vi "Main Page.vi"(8 "error in (no error)":errorcluster, 11 "Node Ptr":T1 format="%.0x") -> (0 "error out":errorcluster)   [LabVIEW 2018, in "Instrument Addon System Explorer.lvlib"]
uses:
  Instrument Addon System Explorer.lvlib
  <vilib>/NI Veristand/Custom Device API/Custom Device Item Ref.ctl
  Addon Shared/Types/FG Control.ctl
  Addon Shared/SubVIs/Constants.vi
  <vilib>/NI/NI VeriStand Advanced SysDef API/SysDef API/SysDef.Property.Get.vi
  <vilib>/NI/NI VeriStand Advanced SysDef API/_SubVIs/SysDef.Property.Get.String.vi
  <vilib>/NI/NI VeriStand Advanced SysDef API/SysDef API/SysDef.Property.Set.vi
  <vilib>/NI/NI VeriStand Advanced SysDef API/_SubVIs/SysDef.Property.Set.String.vi
  <vilib>/Utility/LVClass/Get LV Class Default Value.vi
  Support Libraries/Protocols.lvlibp/TCP/Settings Page.vi
  <vilib>/NI Veristand/Custom Device API/NI VeriStand - Get Item Property.vi
  <vilib>/NI Veristand/Custom Device API/Get Item Property (Boolean).vi
  <vilib>/NI Veristand/Custom Device API/Get Item Property (U32).vi
  <vilib>/NI Veristand/Custom Device API/Get Item Property (String).vi
  <vilib>/NI Veristand/Custom Device API/NI VeriStand - Set Item Property.vi
  <vilib>/NI Veristand/Custom Device API/Set Item Property (Boolean).vi
  <vilib>/NI Veristand/Custom Device API/Set Item Property (U32).vi
  <vilib>/NI Veristand/Custom Device API/Set Item Property (String).vi
  Support Libraries/Protocols.lvlibp/Protocol Parent/Protocol Parent.lvclass
  <vilib>/NI Veristand/Custom Device API/Custom Device API.lvlib
  Addon Shared/Instrument Addon Shared.lvlib
  APIs/Scripting API/Instrument Addon Scripting API.lvlib
  Support Libraries/Protocols.lvlibp/TCP/TCP.lvclass
panel:
  out "Version":string
  in  "PCL Decimation":u32=1 min=1 max=10000 step=1
  in  "Protocol":string(combo)
  in  "SHDocVw.IWebBrowser":refnum<k7>(container)
  in  "Header":cluster{"Section Name":string}={"Section Name"="Addon Settings"}
  in  "Description":string
  in  "Name":string
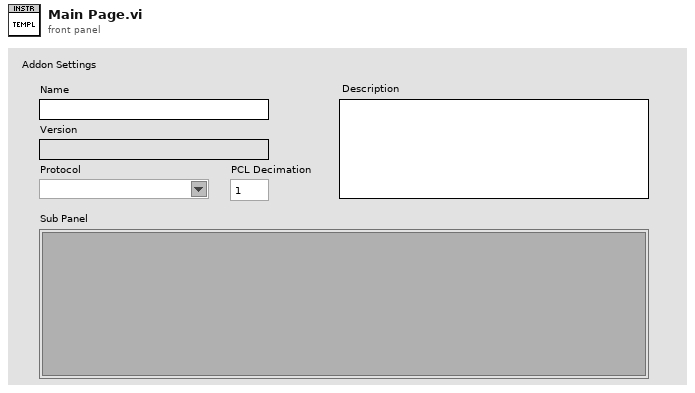
[diagram p1: front panel]
types:
  T1 = typedef "Custom Device API.lvlib/Custom Device Item Ref.ctl" = u64
  T2 = typedef "Custom Device API.lvlib/Custom Device Item Info.ctl" = cluster{"Name":string, "Is Channel":bool, "GUID":string, "Is Waveform":bool}
  T3 = typedef "Instrument Addon Shared.lvlib/FG Control.ctl" = enum16{"Get", "Set"}
  T4 = typedef "Custom Device API.lvlib/Custom Device Commands.ctl" = enum16{"Default", "Item renamed", "Shutdown", "Dynamic button pressed"}
  T5 = typedef "Protocols.lvlibp/Protocol Parent.lvclass/Base Protocol Type.ctl" = enum16{"RS-XXX", "VISA", "TCPIP", "UDP", "GPIB ConvBox"}
  T6 = typedef "Instrument Addon Shared.lvlib/VISA Settings.ctl" = cluster{"VISA Resource":string, "Enable Termination Character":bool, "Termination Character":u8, "Timeout":u32, "Append Write Termination Character":bool}
  T7 = typedef "Instrument Addon Shared.lvlib/TCPIP Settings.ctl" = cluster{"IP Address":string, "Port":u16}
  T8 = typedef "Instrument Addon Shared.lvlib/UDP Settings.ctl" = cluster{"Local IP Address":string, "Local Port":u16, "Target IP Address":string, "Target Port":u16}
  T9 = typedef "Instrument Addon Shared.lvlib/RSXXX Port Settings.ctl" = cluster{"Port":string, "Baud Rate":u32, "Data Bits":u16, "Parity":enum16{"None", "Odd", "Even", "Mark", "Space"}, "Stop Bits":u16, "Flow Control":u16, "XON":enum16{"NUL", "SOH", "STX", "ETX", "EOT", "ENQ", "ACK", "BEL", "BS", "HT", "LF", "VT", "FF", "CR", "SO", "SI", "DLE", "DC1", "DC2", "DC3", "DC4", "NAK", "SYN", "ETB", "CAN", "EM", "SUB", "ESC", "FS", "GS", "RS", "US", "SP", "!", "\"", "#", "$", "%", "&", "'", "(", ")", "*", "+", ",", "- (-)", ".", "/", "0", "1", "2", "3", "4", "5", "6", "7", "8", "9", ":", ";", "<", "=", ">", "?", "@", "A", "B", "C", "D", "E", "F", "G", "H", "I", "J", "K", "L", "M", "N", "O", "P", "Q", "R", "S", "T", "U", "V", "W", "X", "Y", "Z", "[", "\\", "]", "^", "_", "`", "a", "b", "c", "d", "e", "f", "g", "h", "i", "j", "k", "l", "m", "n", "o", "p", "q", "r", "s", "t", "u", "v", "w", "x", "y", "z", "{", "|", "}", "~"}, "XOFF":enum16{"NUL", "SOH", "STX", "ETX", "EOT", "ENQ", "ACK", "BEL", "BS", "HT", "LF", "VT", "FF", "CR", "SO", "SI", "DLE", "DC1", "DC2", "DC3", "DC4", "NAK", "SYN", "ETB", "CAN", "EM", "SUB", "ESC", "FS", "GS", "RS", "US", "SP", "!", "\"", "#", "$", "%", "&", "'", "(", ")", "*", "+", ",", "- (-)", ".", "/", "0", "1", "2", "3", "4", "5", "6", "7", "8", "9", ":", ";", "<", "=", ">", "?", "@", "A", "B", "C", "D", "E", "F", "G", "H", "I", "J", "K", "L", "M", "N", "O", "P", "Q", "R", "S", "T", "U", "V", "W", "X", "Y", "Z", "[", "\\", "]", "^", "_", "`", "a", "b", "c", "d", "e", "f", "g", "h", "i", "j", "k", "l", "m", "n", "o", "p", "q", "r", "s", "t", "u", "v", "w", "x", "y", "z", "{", "|", "}", "~"}, "End Read on Termination Character":bool, "End Write on Termination Character":bool, "Termination Character":u8}
  T10 = enum16{"NUL", "SOH", "STX", "ETX", "EOT", "ENQ", "ACK", "BEL", "BS", "HT", "LF", "VT", "FF", "CR", "SO", "SI", "DLE", "DC1", "DC2", "DC3", "DC4", "NAK", "SYN", "ETB", "CAN", "EM", "SUB", "ESC", "FS", "GS", "RS", "US", "SP", "!", "\"", "#", "$", "%", "&", "'", "(", ")", "*", "+", ",", "- (-)", ".", "/", "0", "1", "2", "3", "4", "5", "6", "7", "8", "9", ":", ";", "<", "=", ">", "?", "@", "A", "B", "C", "D", "E", "F", "G", "H", "I", "J", "K", "L", "M", "N", "O", "P", "Q", "R", "S", "T", "U", "V", "W", "X", "Y", "Z", "[", "\\", "]", "^", "_", "`", "a", "b", "c", "d", "e", "f", "g", "h", "i", "j", "k", "l", "m", "n", "o", "p", "q", "r", "s", "t", "u", "v", "w", "x", "y", "z", "{", "|", "}", "~"}
  T11 = typedef "Instrument Addon Shared.lvlib/GPIB ConvBox Settings.ctl" = cluster{"Port":string, "ConvBox Address":string, "Assert Ren with IFC":bool, "System controller":bool, "IST bit sense":bool, "GPIB Address":string}
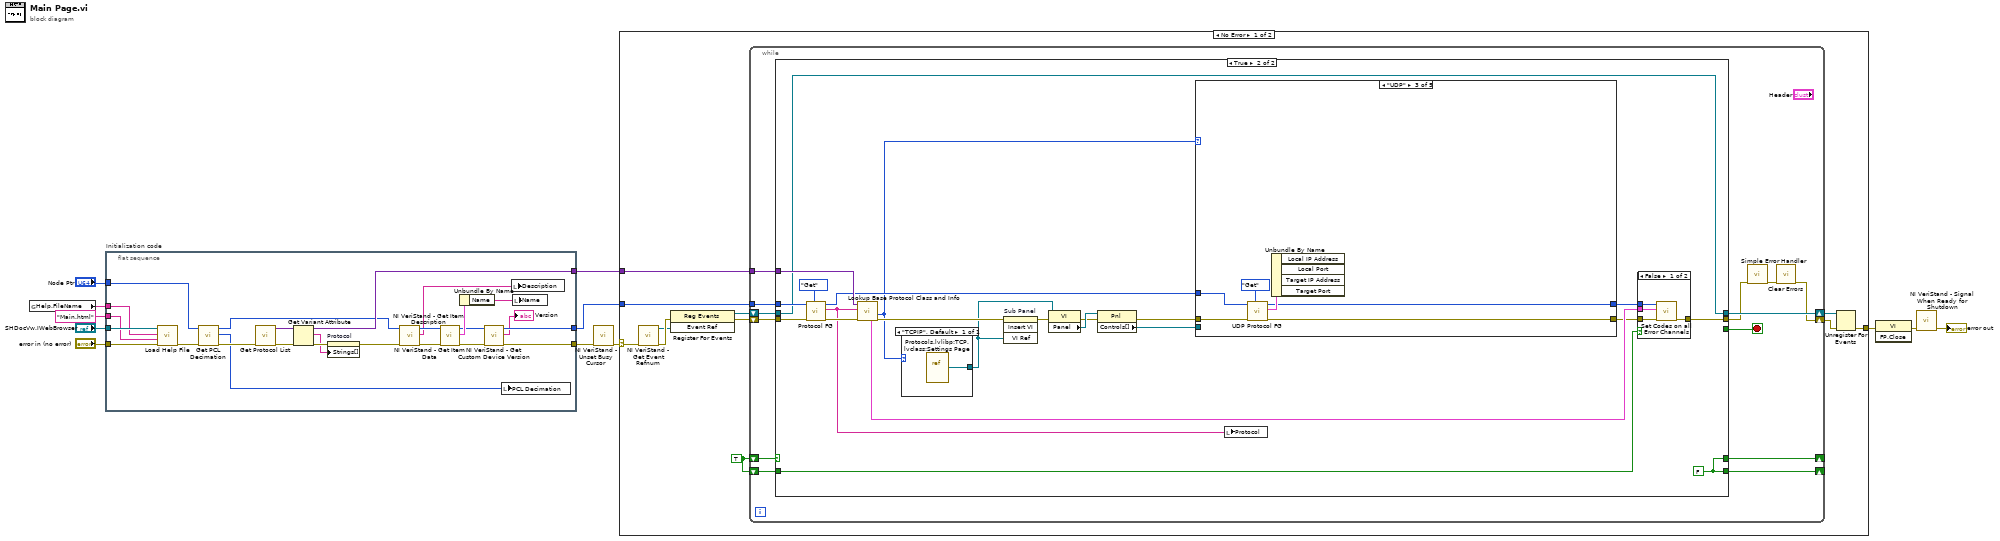
[diagram p0: block diagram]
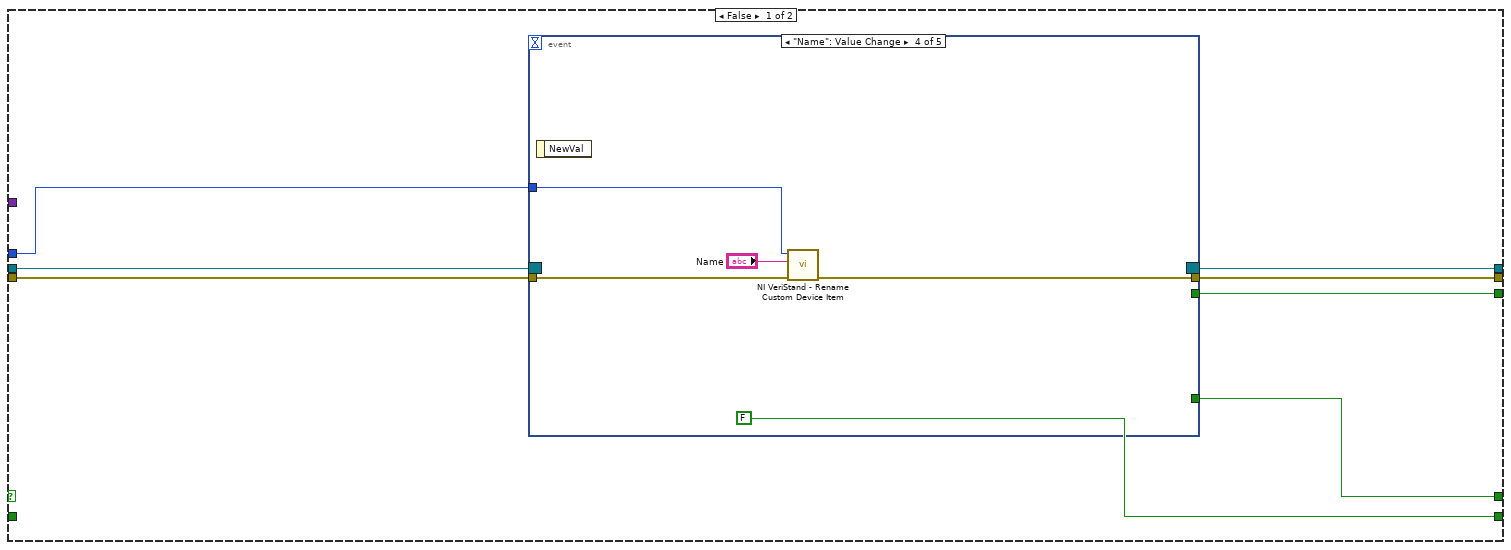
[diagram p2: hidden frame]
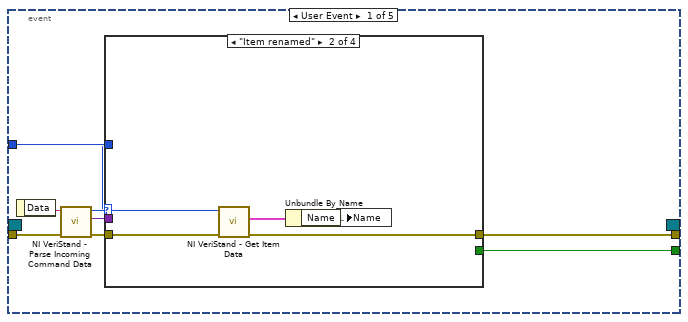
[diagram p3: hidden frame]
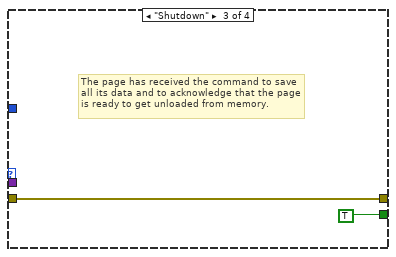
[diagram p5: hidden frame]
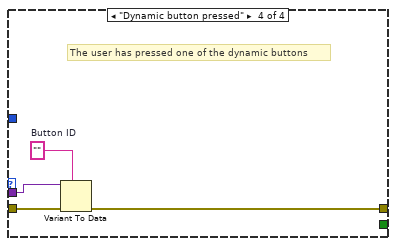
[diagram p6: hidden frame]
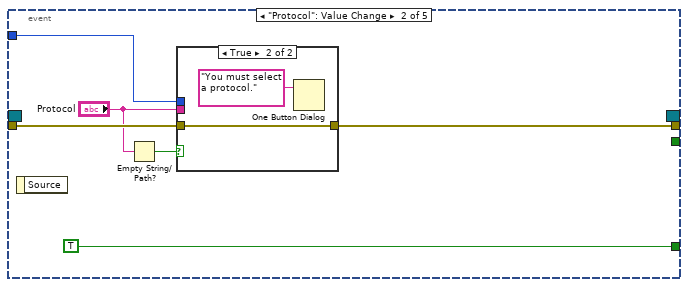
[diagram p7: hidden frame]
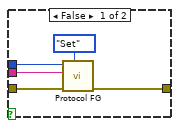
[diagram p8: hidden frame]
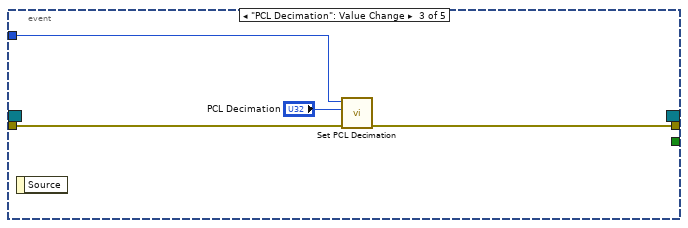
[diagram p9: hidden frame]
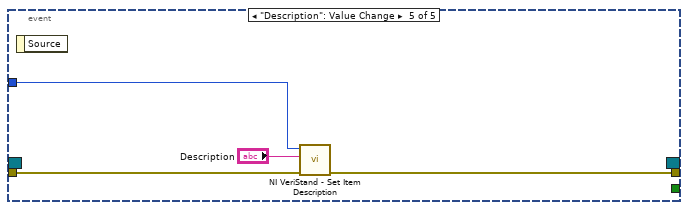
[diagram p10: hidden frame]
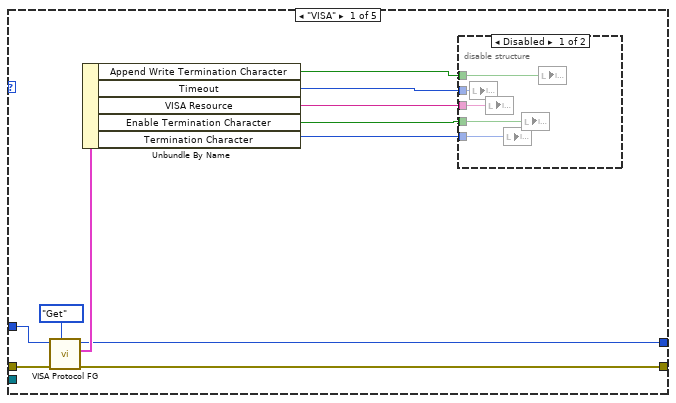
[diagram p12: hidden frame]
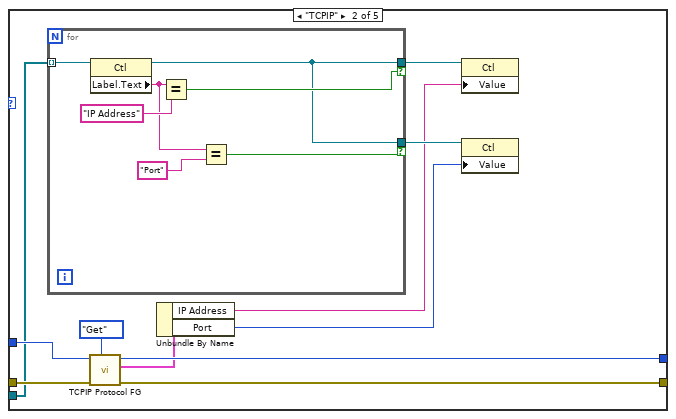
[diagram p14: hidden frame]
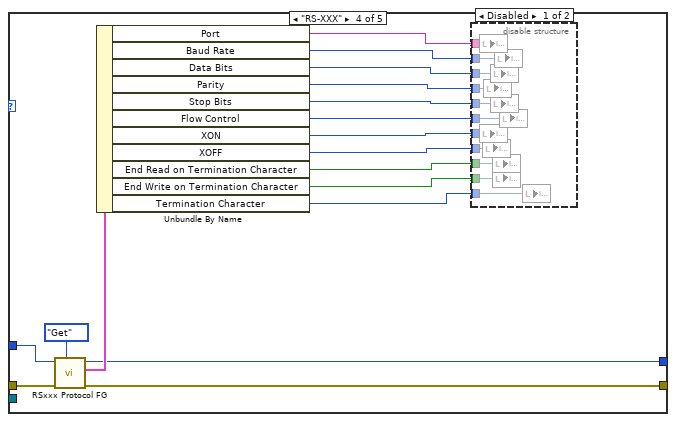
[diagram p15: hidden frame]
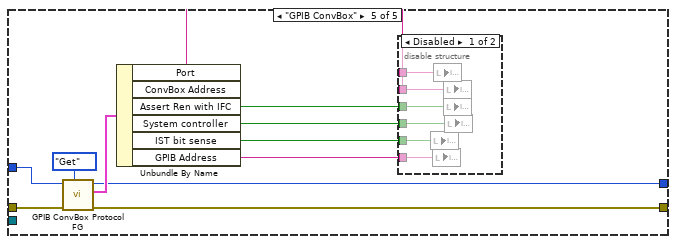
[diagram p17: hidden frame]
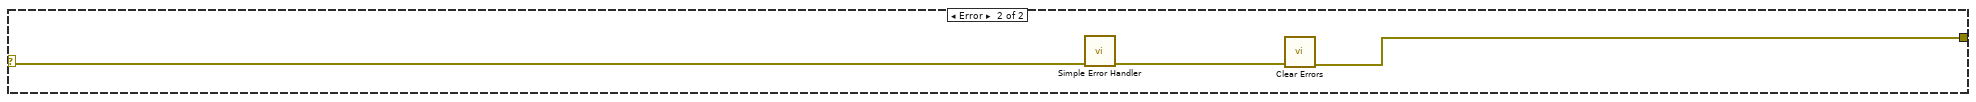
[diagram p19: hidden frame]
diagram:
  n1 = global read "Constants.vi" "Help.FileName"() -> (w1:string)
  n2 = flat-sequence "Initialization code" {
    tunnel: "error in (no error)" -> [w32]
    tunnel: "Node Ptr" -> [w15]
    tunnel: [w21] -> w8
    tunnel: [w19] -> w5
    tunnel: "SHDocVw.IWebBrowser" -> [w31]
    tunnel: "Main.html" ("HTML File") -> [w30]
    tunnel: w1 -> [w29]
    tunnel: [w24] -> w2
    frame #0 {
      n3 = call "Load Help File.vi"("error in (no error)"=w32, "HTML File"=w30, "Main CHM File"=w29, "SHDocVw.IWebBrowser2"=w31) -> ("error out"=w17:errorcluster)  [unwired: 7 in]
      n4 = call "Get PCL Decimation.vi"("Error In"=w17, "Instrument Addon Refnum In"=w15) -> ("Error Out"=w16:errorcluster, "PCL Decimation"=w13:u32, "Instrument Addon Refnum Out"=w14:T1)  [unwired: 7 in]
      n5 = call "Get Protocol List.vi"("error in (no error)"=w16) -> ("error out"=w27:errorcluster, "Class Lookup"=w28:variant)  [unwired: 9 in]
      n6 = Get Variant Attribute(Variant=w28, error in=w27) -> (duplicate Variant=w24:variant, names=w25:string[], error out=w26:errorcluster)  [unwired: 2 in, 1 out]
      n7 = property on="Protocol" class="CmbBox"(error in=w26, "Strings[]"=w25) -> (error out=w23:errorcluster)  [unwired: 1 in, 1 out]
      n8 = call <vilib>:"NI VeriStand - Get Item Description.vi"("error in (no error)"=w23, "Item Ref in"=w14) -> ("error out"=w35:errorcluster, "Description"=w36:string, "Item Ref out"=w37:T1)  [unwired: 7 out]
      n9 = call <vilib>:"NI VeriStand - Get Item Data.vi"("error in (no error)"=w35, "Item Ref in"=w37) -> ("error out"=w22:errorcluster, "Item Info"=w34:T2, "Item Ref out"=w20:T1)  [unwired: 7 out]
      n10 = Unbundle By Name(w34) -> ("Name"=w33:string)
      n11 = call <vilib>:"NI VeriStand - Get Custom Device Version.vi"("error in (no error)"=w22, "Device Ref in"=w20) -> ("error out"=w21:errorcluster, "Value"=→"Version":string, "Device Ref out"=w19:T1)  [unwired: 7 in]
      n12 = local write "PCL Decimation"(w13) -> ()
      n13 = local write "Description"(w36) -> ()
      n14 = local write "Name"(w33) -> ()
    }
  }
  n15 = call <vilib>:"NI VeriStand - Unset Busy Cursor.vi"("error in (no error)"=w8) -> ("error out"=w7:errorcluster)  [unwired: 10 out]
  n16 = case shown="No Error" w7 {
    selector: w7 -> [w40 w231]
    tunnel: [w45 w229] -> w12
    tunnel: w5 -> [w41 _]
    tunnel: w2 -> [w39 _]
    frame No Error {
      w38 = TRUE
      n17 = call <vilib>:"NI VeriStand - Get Event Refnum.vi"("error in (no error)"=w40) -> ("error out"=w48:errorcluster, "Event Ref"=w44:refnum<user-event>)  [unwired: 9 out]
      n18 = register-events(error in=w48, w44) -> (reference out=w42:refnum<event-registration>, error out=w43:errorcluster)  [unwired: 1 in]
      n19 = while {
        tunnel: w41 -> [w57]
        shift-right: [w54] -> w46
        shift-left: w43 -> [w60]
        shift-right: [w61] -> w47
        shift-left: w42 -> [w59]
        tunnel: w39 -> [w53]
        shift-right: [w51] -> _
        shift-left: w38 -> [w52]
        shift-right: [w49] -> _
        shift-left: w38 -> [w50]
        stop <- w58 stop-if-true
        n20 = case shown="True" w52 {
          tunnel: [w69 w129] -> w61
          tunnel: w60 -> [w68 w135]
          tunnel: w59 -> [w67 w129]
          tunnel: [w66 _] -> w58
          tunnel: w57 -> [w65 w134]
          tunnel: [w64 w125] -> w56
          tunnel: w53 -> [_ w133]
          tunnel: [w63 w123] -> w51
          tunnel: w50 -> [_ w124]
          tunnel: [FALSE w123] -> w49
          frame False {
            n21 = event shown="[3] \"Name\": Value Change" {
              selector: w67 -> [_ _ _ _ _]
              dyn-events: [_ _ _ _ _] -> w69
              timeout: _ -> [_ _ _ _ _]
              tunnel: w68 -> [w77 w94 w106 w110 w113]
              tunnel: [w73 _ _ _ _] -> w66
              tunnel: [w72 w90 w105 w109 w112] -> w64
              tunnel: w65 -> [w71 w95 w103 w108 w114]
              tunnel: [_ TRUE _ _ _] -> w63
              event User Event {
                n22 = event-data() -> ("Data"=w76:string)  [unwired: 1 out]
                n23 = call <vilib>:"NI VeriStand - Parse Incoming Command Data.vi"("error in (no error)"=w77, "Incoming data"=w76) -> ("error out"=w75:errorcluster, "Outgoing data"=w70:variant, "Action"=w74:T4)  [unwired: 7 out]
                n24 = case shown="\"Item renamed\"" w74 {
                  tunnel: w75 -> [w78 w83 w84 w89]
                  tunnel: [_ _ TRUE _] -> w73
                  tunnel: [w78 w80 w84 w86] -> w72
                  tunnel: w71 -> [_ w82 _ _]
                  tunnel: w70 -> [_ _ _ w88]
                  frame "Default", Default {
                  }
                  frame "Item renamed" {
                    n25 = call <vilib>:"NI VeriStand - Get Item Data.vi"("error in (no error)"=w83, "Item Ref in"=w82) -> ("error out"=w80:errorcluster, "Item Info"=w81:T2)  [unwired: 8 out]
                    n26 = Unbundle By Name(w81) -> ("Name"=w79:string)
                    n27 = local write "Name"(w79) -> ()
                  }
                  frame "Shutdown" {
                    # "The page has received the command to save all its data and to acknowledge that the page is ready to get unloaded from memory."
                  }
                  frame "Dynamic button pressed" {
                    w87 = ""  # Button ID
                    # "The user has pressed one of the dynamic buttons"
                    n28 = Variant To Data(error in=w89, type=w87, Variant=w88) -> (error out=w86:errorcluster)  [unwired: 1 out]
                  }
                }
              }
              event "Protocol": Value Change {
                n29 = event-data() -> ()  [unwired: 2 out]
                n30 = Empty String/Path?(string/path="Protocol") -> (empty?=w92:bool)
                n31 = case shown="True" w92 {
                  tunnel: w95 -> [w98 _]
                  tunnel: w94 -> [w99 w101]
                  tunnel: [w96 w101] -> w90
                  tunnel: "Protocol" -> [w97 _]
                  frame False {
                    n32 = call "Protocol FG.vi"("Action"=FG_Control."Set", "error in (no error)"=w99, "Protocol"=w97, "Device Item Ref in"=w98) -> ("error out"=w96:errorcluster)  [unwired: 5 in, 2 out]
                  }
                  frame True {
                    n33 = One Button Dialog(message="You must select a protocol.") -> ()  [unwired: 1 in, 1 out]
                  }
                }
              }
              event "PCL Decimation": Value Change {
                n34 = event-data() -> ()  [unwired: 2 out]
                n35 = call "Set PCL Decimation.vi"("Error In"=w106, "PCL Decimation"="PCL Decimation", "Instrument Addon Refnum In"=w103) -> ("Error Out"=w105:errorcluster)  [unwired: 7 in, 1 out]
              }
              event "Name": Value Change {
                n36 = event-data() -> ()  [unwired: 2 out]
                n37 = call <vilib>:"NI VeriStand - Rename Custom Device Item.vi"("error in (no error)"=w110, "New Name"="Name", "Item Ref in"=w108) -> ("error out"=w109:errorcluster)  [unwired: 1 in, 7 out]
              }
              event "Description": Value Change {
                n38 = event-data() -> ()  [unwired: 2 out]
                n39 = call <vilib>:"NI VeriStand - Set Item Description.vi"("error in (no error)"=w113, "Description"="Description", "Item Ref in"=w114) -> ("error out"=w112:errorcluster)  [unwired: 8 out]
              }
            }
          }
          frame True {
            w123 = FALSE
            n40 = call "Protocol FG.vi"("Action"=FG_Control."Get", "error in (no error)"=w135, "Device Item Ref in"=w134) -> ("error out"=w132:errorcluster, "Protocol out"=w130:string, "Item Ref out"=w131:T1)  [unwired: 6 in]
            n41 = call "Lookup Base Protocol Class and Info.vi"("error in (no error)"=w132, "Protocol in"=w130, "Class Lookup"=w133) -> ("error out"=w122:errorcluster, "Protocol out"=w121:T5, "Error Codes"=w128:cluster{"Code":i32, "String":string}[])  [unwired: 4 in, 2 out]
            n42 = case shown="\"TCPIP\", Default" w121 {
              tunnel: [w137] -> w120
              frame "TCPIP", Default {
                n43 = vi-ref "Protocols.lvlibp:TCP.lvclass:Settings Page.vi"() -> (w137:refnum<vi>)
              }
            }
            n44 = invoke on="Sub Panel" class="SubPnl" method="Insert VI"(error in=w122, "VI Ref"=w120) -> (error out=w119:errorcluster)  [unwired: 2 in, 3 out]
            n45 = property class="VI"(reference=w120, error in=w119) -> (error out=w117:errorcluster, "Panel"=w118:refnum<vi>)  [unwired: 1 out]
            n46 = property class="Pnl"(reference=w118, error in=w117) -> (error out=w116:errorcluster, "Controls[]"=w115:refnum<vi>[])  [unwired: 1 out]
            n47 = case shown="\"UDP\"" w121 {
              tunnel: w116 -> [w153 w169 w182 w199 w222]
              tunnel: [w152 w168 w181 w198 w221] -> w126
              tunnel: w131 -> [w151 w167 w180 w197 w220]
              tunnel: [w143 w165 w177 w183 w211] -> w127
              tunnel: w115 -> [_ w164 _ _ _]
              frame "VISA" {
                n48 = call "VISA Protocol FG.vi"("Action"=FG_Control."Get", "error in (no error)"=w153, "Device Item Ref in"=w151) -> ("error out"=w152:errorcluster, "VISA Config"=w149:T6, "Item Ref out"=w143:T1)  [unwired: 6 in]
                n49 = Unbundle By Name(w149) -> ("Append Write Termination Character"=w144:bool, "Timeout"=w145:u32, "VISA Resource"=w148:string, "Enable Termination Character"=w147:bool, "Termination Character"=w146:u8)
                n50 = disable-structure shown="Disabled" {
                  disable-tunnel: w148 -> [w158 _]
                  disable-tunnel: w147 -> [w157 _]
                  disable-tunnel: w146 -> [w156 _]
                  disable-tunnel: w145 -> [w155 _]
                  disable-tunnel: w144 -> [w154 _]
                  frame Disabled {
                    n51 = local write item#-1(w155) -> ()
                    n52 = local write item#-1(w158) -> ()
                    n53 = local write item#-1(w156) -> ()
                    n54 = local write item#-1(w157) -> ()
                    n55 = local write item#-1(w154) -> ()
                  }
                  frame Enabled {
                  }
                }
              }
              frame "TCPIP" {
                n56 = for {
                  tunnel: w164 -> [w176] mode=indexing
                  tunnel: [w173] -> w162 if=w174
                  tunnel: [w173] -> w161 if=w172
                  n57 = property class="Ctl"(reference=w176) -> (reference out=w173:refnum<vi>, "Label.Text"=w171:string)  [unwired: 1 in, 1 out]
                  n58 = Equal?(x=w171, y="IP Address") -> (x = y?=w174:bool)
                  n59 = Equal?(x=w171, y="Port") -> (x = y?=w172:bool)
                }
                n60 = call "TCPIP Protocol FG.vi"("Action"=FG_Control."Get", "error in (no error)"=w169, "Device Item Ref in"=w167) -> ("error out"=w168:errorcluster, "TCP/IP Config"=w163:T7, "Item Ref out"=w165:T1)  [unwired: 6 in]
                n61 = Unbundle By Name(w163) -> ("IP Address"=w160:string, "Port"=w159:u16)
                n62 = property class="Ctl"(reference=w162, "Value"=w160) -> ()  [unwired: 1 in, 2 out]
                n63 = property class="Ctl"(reference=w161, "Value"=w159) -> ()  [unwired: 1 in, 2 out]
              }
              frame "UDP" {
                n64 = call "UDP Protocol FG.vi"("Action"=FG_Control."Get", "error in (no error)"=w182, "Device Item Ref in"=w180) -> ("error out"=w181:errorcluster, "UDP Config"=w178:T8, "Item Ref out"=w177:T1)  [unwired: 6 in]
                n65 = Unbundle By Name(w178) -> ()  [unwired: 4 out]
              }
              frame "RS-XXX" {
                n66 = call "RSxxx Protocol FG.vi"("Action"=FG_Control."Get", "error in (no error)"=w199, "Device Item Ref in"=w197) -> ("error out"=w198:errorcluster, "Serial Config"=w195:T9, "Item Ref out"=w183:T1)  [unwired: 6 in]
                n67 = Unbundle By Name(w195) -> ("Port"=w194:string, "Baud Rate"=w193:u32, "Data Bits"=w184:u16, "Parity"=w185:enum16{"None", "Odd", "Even", "Mark", "Space"}, "Stop Bits"=w186:u16, "Flow Control"=w187:u16, "XON"=w188:T10, "XOFF"=w189:T10, "End Read on Termination Character"=w190:bool, "End Write on Termination Character"=w191:bool, "Termination Character"=w192:u8)
                n68 = disable-structure shown="Disabled" {
                  disable-tunnel: w194 -> [w210 _]
                  disable-tunnel: w193 -> [w209 _]
                  disable-tunnel: w192 -> [w208 _]
                  disable-tunnel: w191 -> [w207 _]
                  disable-tunnel: w190 -> [w206 _]
                  disable-tunnel: w189 -> [w205 _]
                  disable-tunnel: w188 -> [w204 _]
                  disable-tunnel: w187 -> [w203 _]
                  disable-tunnel: w186 -> [w202 _]
                  disable-tunnel: w185 -> [w201 _]
                  disable-tunnel: w184 -> [w200 _]
                  frame Disabled {
                    n69 = local write item#-1(w210) -> ()
                    n70 = local write item#-1(w204) -> ()
                    n71 = local write item#-1(w205) -> ()
                    n72 = local write item#-1(w201) -> ()
                    n73 = local write item#-1(w200) -> ()
                    n74 = local write item#-1(w202) -> ()
                    n75 = local write item#-1(w206) -> ()
                    n76 = local write item#-1(w207) -> ()
                    n77 = local write item#-1(w209) -> ()
                    n78 = local write item#-1(w203) -> ()
                    n79 = local write item#-1(w208) -> ()
                  }
                  frame Enabled {
                  }
                }
              }
              frame "GPIB ConvBox" {
                n80 = call "GPIB ConvBox Protocol FG.vi"("Action"=FG_Control."Get", "error in (no error)"=w222, "Device Item Ref in"=w220) -> ("error out"=w221:errorcluster, "GPIB ConvBox Config"=w218:T11, "Item Ref out"=w211:T1)  [unwired: 6 in]
                n81 = Unbundle By Name(w218) -> ("Port"=w217:string, "ConvBox Address"=w216:string, "Assert Ren with IFC"=w215:bool, "System controller"=w214:bool, "IST bit sense"=w213:bool, "GPIB Address"=w212:string)
                n82 = disable-structure shown="Disabled" {
                  disable-tunnel: w217 -> [w228 _]
                  disable-tunnel: w216 -> [w227 _]
                  disable-tunnel: w215 -> [w226 _]
                  disable-tunnel: w214 -> [w225 _]
                  disable-tunnel: w213 -> [w224 _]
                  disable-tunnel: w212 -> [w223 _]
                  frame Disabled {
                    n83 = local write item#-1(w224) -> ()
                    n84 = local write item#-1(w223) -> ()
                    n85 = local write item#-1(w228) -> ()
                    n86 = local write item#-1(w227) -> ()
                    n87 = local write item#-1(w226) -> ()
                    n88 = local write item#-1(w225) -> ()
                  }
                  frame Enabled {
                  }
                }
              }
            }
            n89 = local write "Protocol"(w130) -> ()
            n90 = case shown="False" w124 {
              tunnel: w128 -> [w141 _]
              tunnel: w127 -> [w140 _]
              tunnel: w126 -> [w139 w142]
              tunnel: [w138 w142] -> w125
              frame False {
                n91 = call "Set Codes on all Error Channels.vi"("error in (no error)"=w139, "Error Codes"=w141, "Node Ptr in"=w140) -> ("error out"=w138:errorcluster)  [unwired: 7 in, 1 out]
              }
              frame True {
              }
            }
          }
        }
        n92 = call <vilib>:"Simple Error Handler.vi"("error in (no error)"=w56) -> ("error out"=w55:errorcluster)  [unwired: 1 in, 7 out]
        n93 = call <vilib>:"Clear Errors.vi"("error in (no error)"=w55) -> ("error out"=w54:errorcluster)  [unwired: 1 in, 5 out]
      }
      n94 = Unregister For Events(event registration refnum=w47, error in=w46) -> (error out=w45:errorcluster)
    }
    frame Error {
      n95 = call <vilib>:"Simple Error Handler.vi"("error in (no error)"=w231) -> ("error out"=w230:errorcluster)  [unwired: 1 in, 7 out]
      n96 = call <vilib>:"Clear Errors.vi"("error in (no error)"=w230) -> ("error out"=w229:errorcluster)  [unwired: 1 in, 5 out]
    }
  }
  n97 = invoke class="VI" method="FP.Close"(error in=w12) -> (error out=w11:errorcluster)  [unwired: 2 in, 2 out]
  n98 = call <vilib>:"NI VeriStand - Signal When Ready for Shutdown.vi"("error in (no error)"=w11) -> ("error out"=→"error out":errorcluster)  [unwired: 10 out]
